vi "Add Resource (Equalization).vi"(0 "instance":u8, 1 "number of filter coefficients":u8, 2 "gen in":refnum<class "niUSRP Tx DSP v2 FPGA.lvclass">, 3 "collection builder in":refnum<class "Collection Builder.lvclass">, 5 "IP enabled":bool, 7 "overclock":refnum<k21>, 9 "overclock factor":u8, 11 "filter type":T1, 12 "channel":u8) -> (13 "gen out":refnum<class "niUSRP Tx DSP v2 FPGA.lvclass">, 14 "collection builder out":refnum<class "Collection Builder.lvclass">)   [LabVIEW 2025, in "niUSRP Tx DSP v2 FPGA.lvclass"]
uses:
  niUSRP Tx DSP v2 FPGA.lvclass
  <instrlib>/_niInstr/Instruction Framework/v1/FPGA/Collection Builder/Collection Builder.lvclass
  <instrlib>/_niInstr/DSP Control/Common/v2/FPGA/Equalization/Registers/Equalization Filter Type.ctl
  <instrlib>/_niInstr/DSP Control/Interface/v1/FPGA/Equalization/IQ 18-bit/Equalization Interface (IQ 18-bit).lvclass
  <instrlib>/_niInstr/DSP Control/Interface/v1/FPGA/Equalization/Programming/EQ Programming Interface.lvclass
  <instrlib>/_niInstr/DSP Control/Common/v2/FPGA/Equalization/EQ FIFO/EQ FIFO.lvclass
  C:/Program Files/NI/LVAddons/niidl/1/instr.lib/_niInstr/DSP Control/Interface/v1/FPGA/Equalization/Programming/EQ Programming Interface.lvclass
  <instrlib>/_niInstr/DSP Control/Common/v2/FPGA/Equalization/IQ 18-bit/Equalization (IQ 18-bit).lvclass
  C:/Program Files/NI/LVAddons/niidl/1/instr.lib/_niInstr/DSP Control/Interface/v1/FPGA/Equalization/IQ 18-bit/Equalization Interface (IQ 18-bit).lvclass
  <instrlib>/_niInstr/Instruction Framework/v1/FPGA/Helper Classes/Single Address Space Collection/Single Address Space Collection.lvclass
  C:/Program Files/NI/LVAddons/niidl/1/instr.lib/_niInstr/Instruction Framework/v1/FPGA/Interfaces/Address Space Collection/Address Space Collection.lvclass
  <instrlib>/_niInstr/Basic Elements/v1/FPGA/niInstr Basic Elements v1 FPGA.lvlib
  <instrlib>/_niInstr/DSP Control/Common/v2/FPGA/Equalization/Registers/Equalization Registers.lvclass
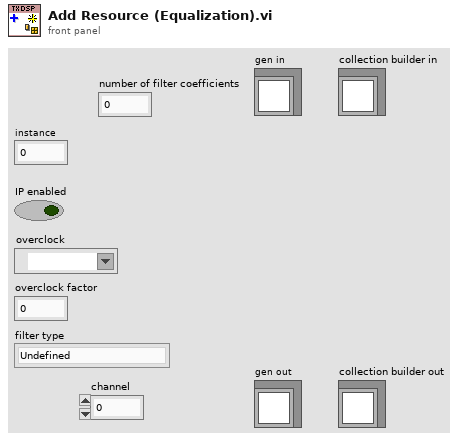
[diagram p1: front panel]
types:
  T1 = typedef "niInstr DSP Control Common v2 FPGA.lvlib/Equalization Registers.lvclass/Equalization Filter Type.ctl" = enum8{"Undefined", "Single", "Complex", "Matrix"}
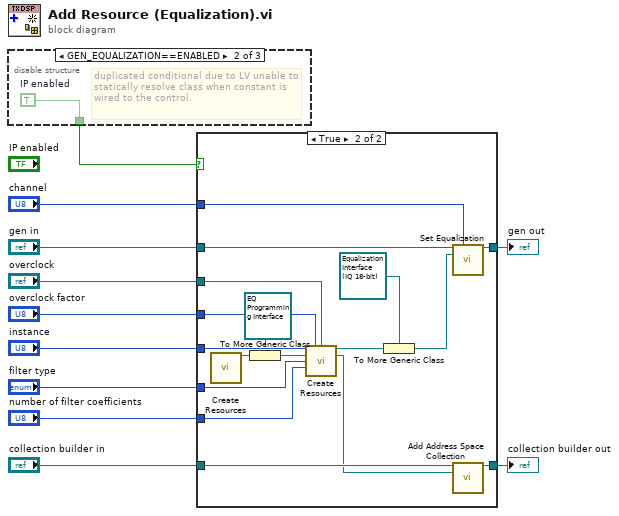
[diagram p0: block diagram]
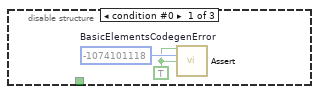
[diagram p2: hidden frame]
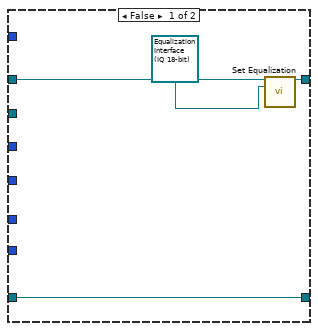
[diagram p4: hidden frame]
diagram:
  n1 = disable-structure shown="GEN_EQUALIZATION==ENABLED" {
    disable-tunnel: [_ w14 _] -> w3
    frame condition #0 {
      w12 = TRUE ("assert")
      w13 = -1074101118  # BasicElementsCodegenError
      n2 = call <instrlib>:"Assert.vi"("assert"=w12, "error code"=w13, "enable show error"=w12) -> ()  [unwired: 13 in]
    }
    frame condition #1 {
      w14 = TRUE  # IP enabled
      # "duplicated conditional due to LV unable to statically resolve class when constant is wired to the control."
    }
    frame condition #2 (active) {
    }
  }
  n3 = case shown="True" w3 {
    tunnel: "collection builder in" -> [w18 w35]
    tunnel: [w18 w34] -> w10
    tunnel: "instance" -> [_ w32]
    tunnel: "gen in" -> [w16 w27]
    tunnel: [w15 w26] -> w7
    tunnel: "number of filter coefficients" -> [_ w21]
    tunnel: "overclock factor" -> [_ w29]
    tunnel: "overclock" -> [_ w28]
    tunnel: "filter type" -> [_ w20]
    tunnel: "channel" -> [_ w19]
    frame False {
      n4 = call-dynamic "Set Equalization.vi"("gen in"=w16, "equalization"=refnum<class "Equalization Interface (IQ 18-bit).lvclass"> refnum) -> ("gen out"=w15:refnum<class "niUSRP Tx DSP v2 FPGA.lvclass">)  [unwired: 13 in]
    }
    frame True {
      n5 = call <instrlib>:"Create Resources.vi"() -> ("EQ FIFO"=w24:refnum<class "EQ FIFO.lvclass">)  [unwired: 15 in]
      n6 = To More Generic Class(target class=refnum<class "EQ Programming Interface.lvclass"> refnum ("niInstr DSP Control Interface v1 FPGA.lvlib:EQ Programming Interface.lvclass"), reference=w24) -> (generic class reference=w23:refnum<class "EQ Programming Interface.lvclass">)
      n7 = call <instrlib>:"Create Resources.vi"("instance"=w32, "overclock factor"=w29, "overclock"=w28, "EQ Programming channel"=w23, "filter type"=w20, "number of filter coefficients"=w21) -> ("equalization"=w31:refnum<class "Equalization (IQ 18-bit).lvclass">, "equalization registers"=w30:refnum<class "Single Address Space Collection.lvclass">)  [unwired: 8 in]
      n8 = To More Generic Class(target class=refnum<class "Equalization Interface (IQ 18-bit).lvclass"> refnum ("equalization"), reference=w31) -> (generic class reference=w25:refnum<class "Equalization Interface (IQ 18-bit).lvclass">)
      n9 = call-dynamic "Set Equalization.vi"("gen in"=w27, "channel"=w19, "equalization"=w25) -> ("gen out"=w26:refnum<class "niUSRP Tx DSP v2 FPGA.lvclass">)  [unwired: 12 in]
      n10 = call <instrlib>:"Add Address Space Collection.vi"("collection builder in"=w35, "address space collection"=w30) -> ("collection builder out"=w34:refnum<class "Collection Builder.lvclass">)  [unwired: 13 in]
    }
  }
  "collection builder out" <- w10
  "gen out" <- w7
